vi "DriveDual.vi"(9 "YAxis":dbl, 10 "XAxis":dbl, 11 "Turbo?":bool) -> (2 "Right":dbl, 3 "Left":dbl)   [LabVIEW 2018]
uses:
  <vilib>/Rock Robotics/Network Tables/NT Write Boolean.vi
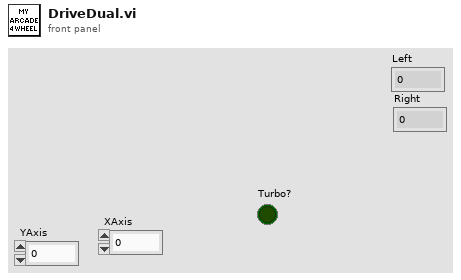
[diagram p1: front panel]
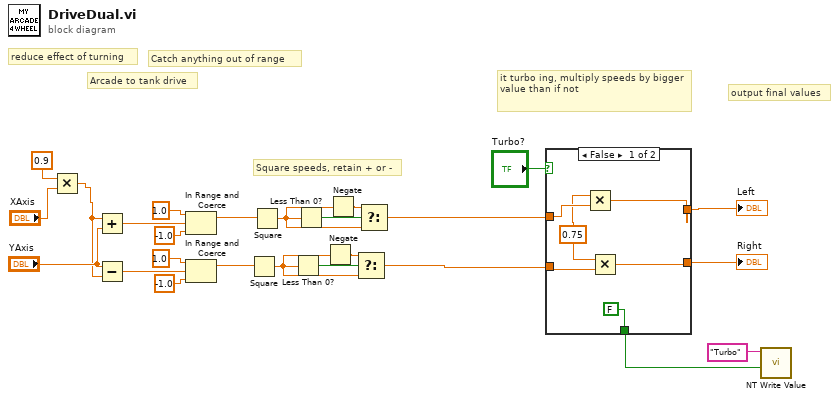
[diagram p0: block diagram]
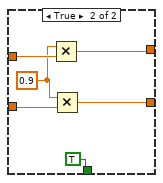
[diagram p2: hidden frame]
diagram:
  # "output final values"
  # "it turbo ing, multiply speeds by bigger value than if not"
  # "Catch anything out of range"
  # "Arcade to tank drive"
  # "reduce effect of turning"
  # "Square speeds, retain + or -"
  n1 = Multiply(x=0.9, y="XAxis") -> (x*y=w11:dbl)
  n2 = Add(x=w11, y="YAxis") -> (x+y=w25:dbl)
  n3 = Subtract(x="YAxis", y=w11) -> (x-y=w20:dbl)
  n4 = In Range and Coerce(upper limit=1.0, x=w25, lower limit=-1.0) -> (coerced(x)=w8:dbl)  [unwired: 1 out]
  n5 = In Range and Coerce(upper limit=1.0, x=w20, lower limit=-1.0) -> (coerced(x)=w2:dbl)  [unwired: 1 out]
  n6 = Square(x=w2) -> (x^2=w6:dbl)
  n7 = Square(x=w8) -> (x^2=w7:dbl)
  n8 = Less Than 0?(x=w6) -> (x < 0?=w4:bool)
  n9 = Less Than 0?(x=w7) -> (x < 0?=w19:bool)
  n10 = Negate(x=w6) -> (-x=w5:dbl)
  n11 = Negate(x=w7) -> (-x=w18:dbl)
  n12 = Select(t=w5, s=w4, f=w6) -> (s? t:f=w3:dbl)
  n13 = Select(t=w18, s=w19, f=w7) -> (s? t:f=w16:dbl)
  n14 = case shown="False" "Turbo?" {
    tunnel: w16 -> [w31 w36]
    tunnel: [w30 w35] -> w15
    tunnel: w3 -> [w29 w33]
    tunnel: [w28 w34] -> w14
    tunnel: [FALSE TRUE] -> w9
    frame False {
      w26 = 0.75
      n15 = Multiply(x=w26, y=w31) -> (x*y=w30:dbl)
      n16 = Multiply(x=w26, y=w29) -> (x*y=w28:dbl)
    }
    frame True {
      w32 = 0.9
      n17 = Multiply(x=w32, y=w36) -> (x*y=w35:dbl)
      n18 = Multiply(x=w32, y=w33) -> (x*y=w34:dbl)
    }
  }
  "Left" <- w15
  "Right" <- w14
  n19 = call-poly <vilib>:"NT Write Value.vi"("Boolean"=w9, "Name"="Turbo") -> ()  [unwired: 9 in, 1 out]
